vi "DBM inquiry.vi"(6 "컨트롤 참조":refnum<vi>[](array[refnum]), 7 "Query info":T2, 8 "에러 입력":errorcluster caption="에러 입력(에러 없음)", 11 "데이터":T1) -> (0 "에러 출력":errorcluster, 1 "None?":bool, 2 "Data":string[][](array[string]), 3 "테이블 참조 출력":refnum<vi>, 5 "데이터 out":T1)   [LabVIEW 2020]
uses:
  Controls/Clst_DBM data.ctl
  Controls/Clst_Query Info.ctl
  Controls/Cmd_Read Query.ctl
  <vilib>/addons/database/NI_Database_API.lvlib
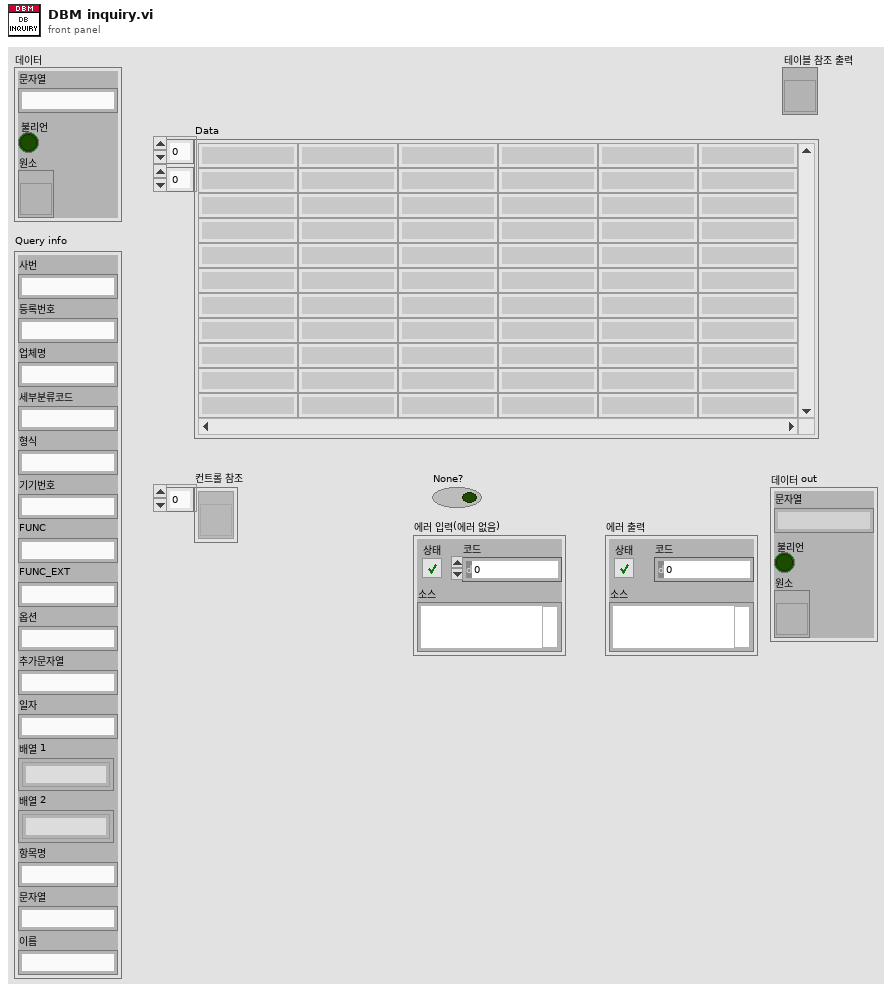
[diagram p1: front panel]
types:
  T1 = typedef "Clst_DBM data.ctl" = cluster{"문자열":string, "불리언":bool, "원소":refnum<vi>}
  T2 = typedef "Clst_Query Info.ctl" = cluster{"사번":string, "등록번호":string, "업체명":string, "세부분류코드":string, "형식":string, "기기번호":string, "FUNC":string, "FUNC_EXT":string, "옵션":string, "추가문자열":string, "일자":string, "배열 1":string[], "배열 2":string[], "항목명":string, "문자열":string, "이름":string}
  T3 = typedef "Cmd_Read Query.ctl" = enum16{"교정자 이름 얻기", "인증교정자 얻기", "기술책임자 얻기", "기책부책 얻기", "등록번호 얻기", "등록정보 얻기", "업체정보 얻기", "교정일자(CAMAS) 얻기", "교정일자(CALSTD) 얻기", "교정환경 얻기", "교정절차서 목록 얻기", "교정절차서명 얻기", "교정절차 목록얻기", "교정절차 얻기", "PROC 교정절차 얻기", "PROC SPEC 얻기", "교정절차(Func별) 얻기", "교정절차(Func_ext별) 얻기", "기관코드 얻기", "교정기능(세부분류) 얻기", "교정기능(모델) 얻기", "교정기능 목록 얻기", "교정기능 명칭 얻기", "교정기능 항목명칭 얻기", "DB (사용기준기) 얻기", "DB (기준기이름) 얻기", "DB (기준기이름목록) 얻기", "DB (기준기목록) 얻기", "DB (기준기값) 얻기", "DB (CMC) 얻기", "DB (FUNC) 얻기", "DB (CALNAME) 얻기", "DB (STDNAME) 얻기", "DB (SPEC) 얻기", "모델(항목전체) 얻기", "모델(최대범위) 얻기", "모델(최소범위) 얻기", "모델(최대최소) 얻기", "모델(범위조건) 얻기", "모델(등록요청) 얻기", "모델(형식별) 얻기", "모델(조건별) 얻기", "모델(모델검색) 얻기", "세부분류 목록 얻기", "기준기등록리스트 얻기", "STD Cal Date Check", "DB등록일자 얻기", "적용항목 얻기", "기타정보 얻기", "기준기요청 얻기", "서버버전 얻기"}
  T4 = typedef "NI_Database_API.lvlib/Conn ObjectReference.ctl" = refnum<k1>
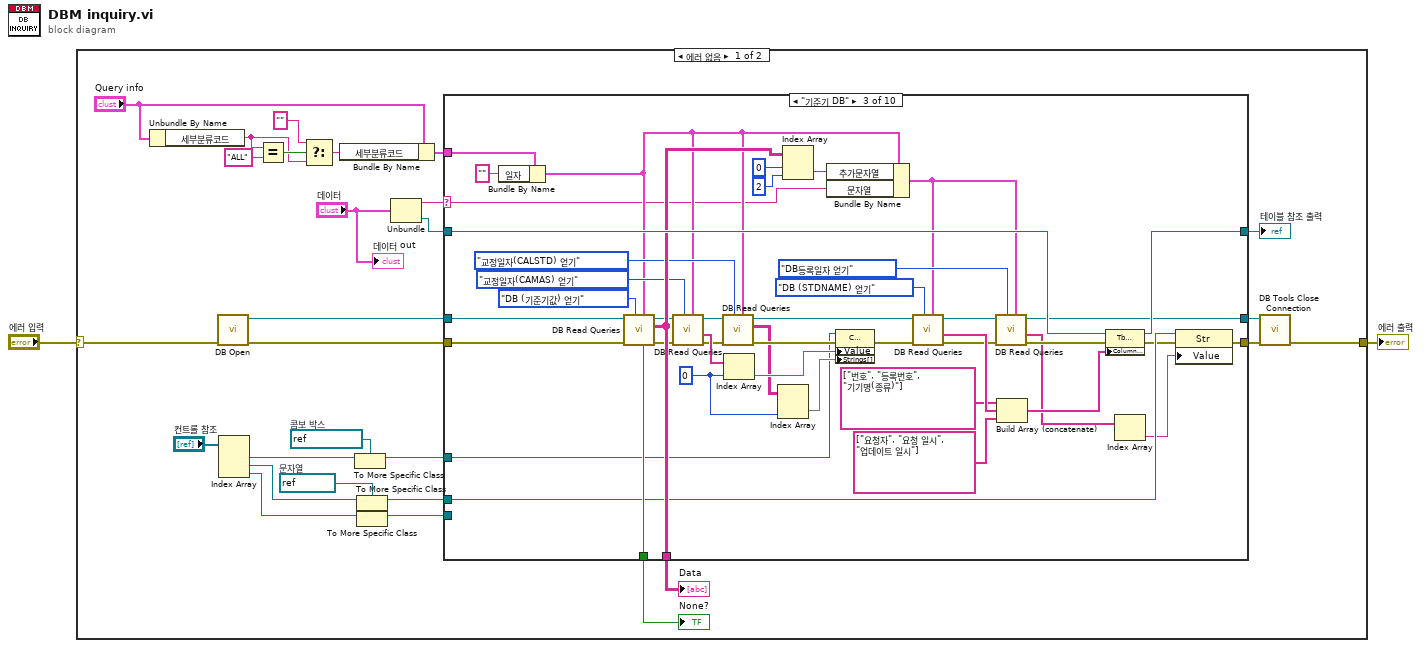
[diagram p0: block diagram]
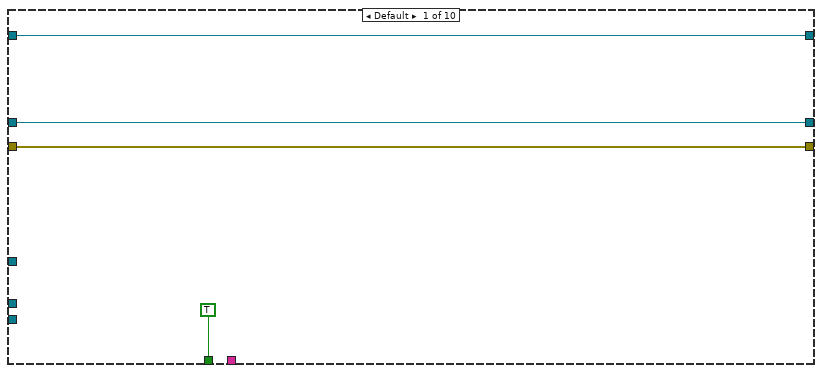
[diagram p2: hidden frame]
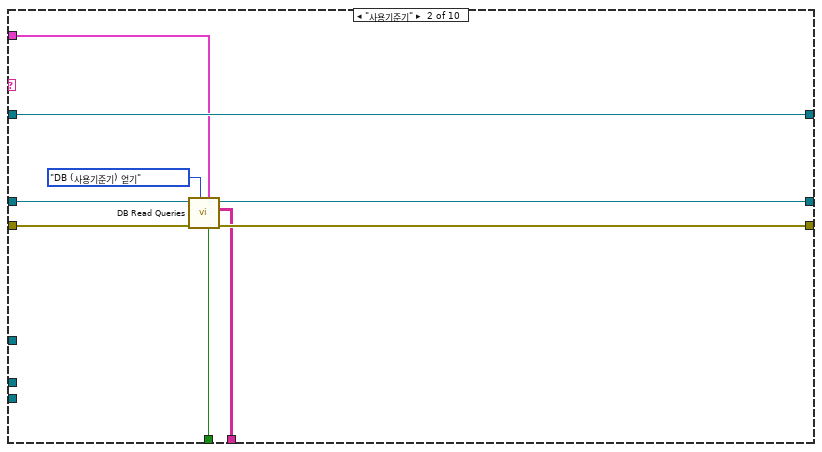
[diagram p3: hidden frame]
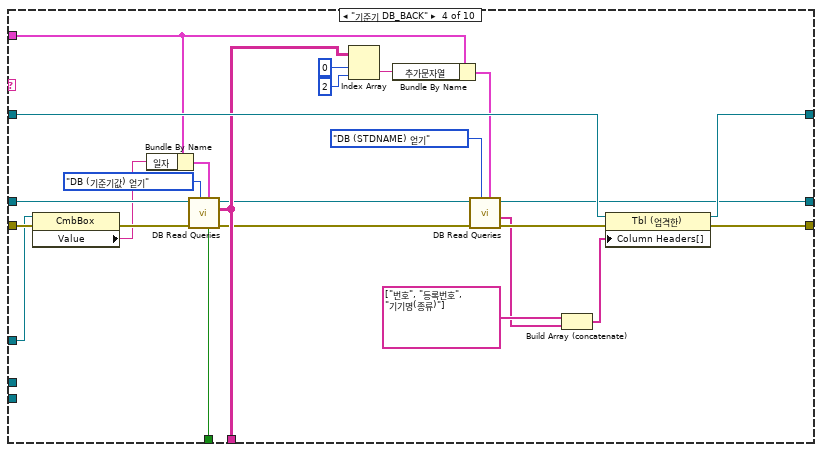
[diagram p4: hidden frame]
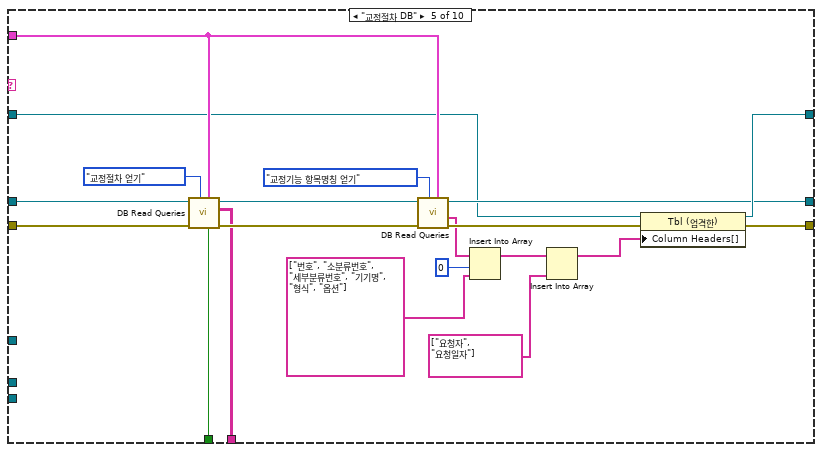
[diagram p5: hidden frame]
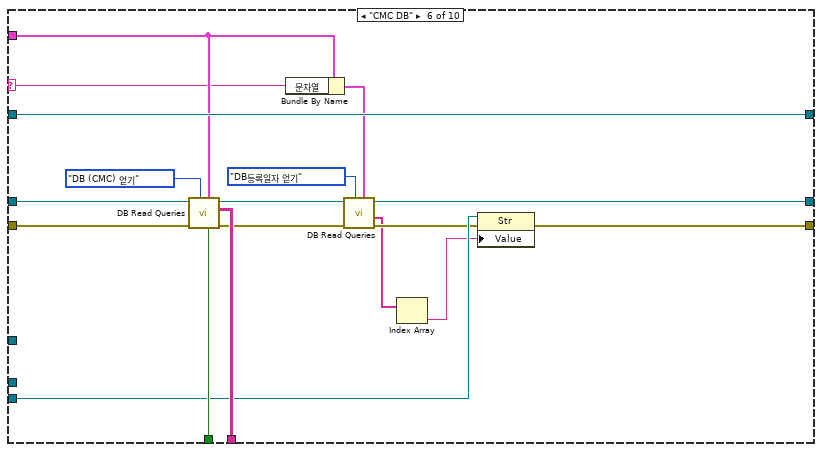
[diagram p6: hidden frame]
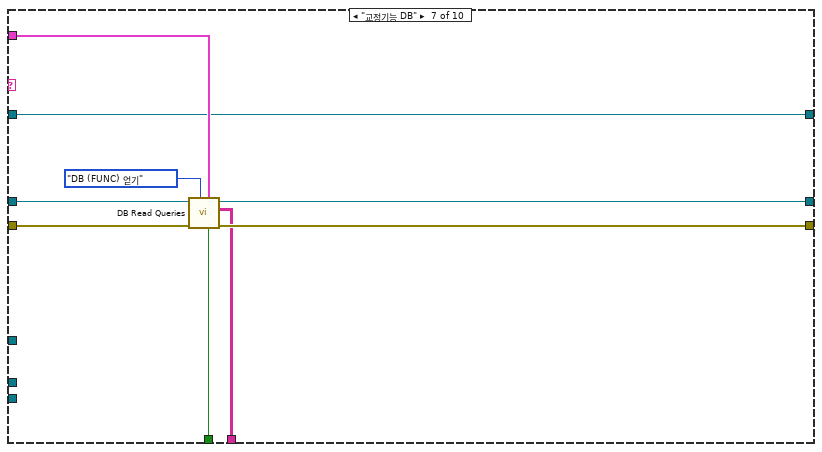
[diagram p7: hidden frame]
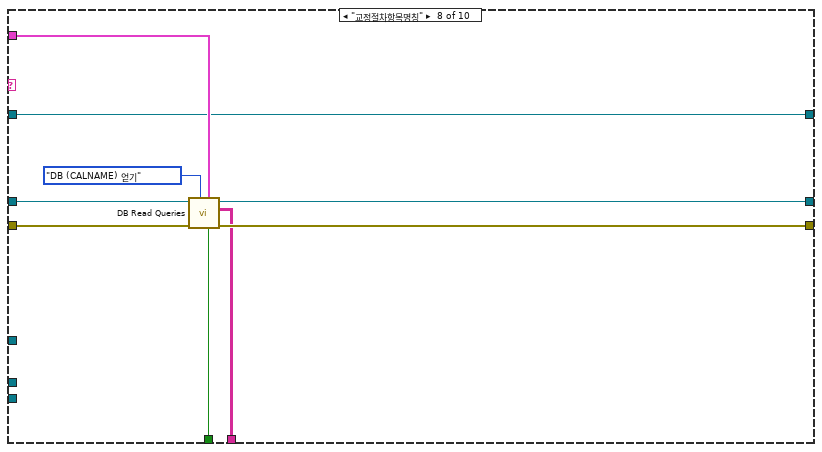
[diagram p8: hidden frame]
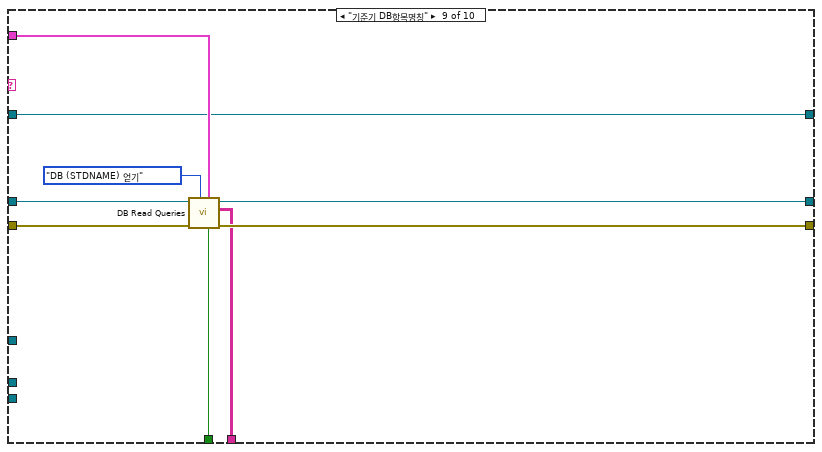
[diagram p9: hidden frame]
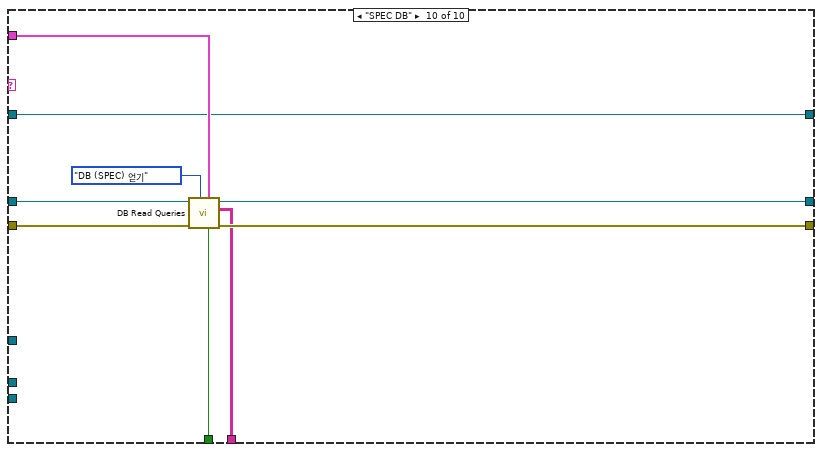
[diagram p10: hidden frame]
diagram:
  n1 = case shown="에러 없음" "에러 입력" {
    selector: "에러 입력" -> [w17 w187]
    tunnel: [w19 w187] -> w2
    frame No Error {
      w10 = refnum<vi> refnum  # 문자열
      w13 = refnum<vi> refnum  # 콤보 박스
      n2 = Unbundle By Name("Query info") -> ("세부분류코드"=w27:string)
      n3 = call "DB Open.vi"("에러 입력"=w17) -> ("에러 출력"=w22:errorcluster, "참조 번호 출력"=w21:T4)  [unwired: 9 in]
      n4 = Index Array(array="컨트롤 참조") -> (element #1=w15:refnum<vi>, element #2=w12:refnum<vi>, element #3=w9:refnum<vi>)  [unwired: 3 in]
      n5 = Equal?(x=w27, y="ALL") -> (x = y?=w28:bool)
      n6 = Select(t="", s=w28, f=w27) -> (s? t:f=w26:string)
      n7 = Bundle By Name(cluster="Query info", "세부분류코드"=w26) -> (w23:T2)
      n8 = To More Specific Class(target class=w13, reference=w15) -> (specific class reference=w14:refnum<vi>)  [unwired: 1 in, 1 out]
      n9 = To More Specific Class(target class=w10, reference=w12) -> (specific class reference=w11:refnum<vi>)  [unwired: 1 in, 1 out]
      n10 = To More Specific Class(target class=w10, reference=w9) -> (specific class reference=w8:refnum<vi>)  [unwired: 1 in, 1 out]
      n11 = Unbundle("데이터") -> ("문자열"=w5:string, "원소"=w3:refnum<vi>)  [unwired: 1 out]
      n12 = case shown="\"기준기 DB\"" w5 {
        selector: w5 -> [_ _ w46 _ _ w135 _ _ _ _]
        tunnel: [TRUE ("None?") w42 w87 w112 w131 w149 w158 w167 w176 w185] -> w30
        tunnel: w22 -> [w34 w41 w86 w92 w130 w148 w157 w166 w175 w184]
        tunnel: [w34 w40 w47 w111 w128 w143 w156 w165 w174 w183] -> w20
        tunnel: [_ w39 w81 w103 w127 w147 w155 w164 w173 w182] -> w24
        tunnel: [w32 w37 w85 w110 w126 w146 w152 w161 w170 w179] -> w7
        tunnel: w23 -> [_ w35 w60 w94 w124 w137 w154 w163 w172 w181]
        tunnel: [w33 w38 w54 w107 w123 w139 w153 w162 w171 w180] -> w18
        tunnel: w3 -> [w32 w37 w84 w109 w122 w146 w152 w161 w170 w179]
        tunnel: w21 -> [w33 w36 w83 w108 w121 w145 w151 w160 w169 w178]
        tunnel: w14 -> [_ _ w50 w90 _ _ _ _ _ _]
        tunnel: w11 -> [_ _ w49 _ _ _ _ _ _ _]
        tunnel: w8 -> [_ _ _ _ _ w144 _ _ _ _]
        frame Default {
        }
        frame "사용기준기" {
          n13 = call "DB Read Queries.vi"("Query info"=w35, "Query Command"=Cmd_Read_Query."DB (사용기준기) 얻기", "에러 입력(에러 없음)"=w41, "참조 번호 입력"=w36) -> ("에러 출력"=w40:errorcluster, "Data"=w39:string[][], "참조 번호 출력"=w38:T4, "None?"=w42:bool)  [unwired: 3 in, 1 out]
        }
        frame "기준기 DB" {
          w62 = 0 ("인덱스 (행)")
          n14 = Bundle By Name(cluster=w60, "일자"="") -> (w58:T2)
          n15 = call "DB Read Queries.vi"("Query info"=w58, "Query Command"=Cmd_Read_Query."DB (기준기값) 얻기", "에러 입력(에러 없음)"=w86, "참조 번호 입력"=w83) -> ("에러 출력"=w75:errorcluster, "Data"=w81:string[][], "참조 번호 출력"=w76:T4, "None?"=w87:bool)  [unwired: 3 in, 1 out]
          n16 = call "DB Read Queries.vi"("Query info"=w58, "Query Command"=Cmd_Read_Query."교정일자(CAMAS) 얻기", "에러 입력(에러 없음)"=w75, "참조 번호 입력"=w76) -> ("에러 출력"=w68:errorcluster, "Data (0번행)"=w74:string[], "참조 번호 출력"=w66:T4)  [unwired: 3 in, 2 out]
          n17 = call "DB Read Queries.vi"("Query info"=w58, "Query Command"=Cmd_Read_Query."교정일자(CALSTD) 얻기", "에러 입력(에러 없음)"=w68, "참조 번호 입력"=w66) -> ("에러 출력"=w67:errorcluster, "Data"=w63:string[][], "참조 번호 출력"=w65:T4)  [unwired: 3 in, 2 out]
          n18 = Index Array(array=w74, index=w62) -> (element=w71:string)
          n19 = Index Array(array=w63, index (col)=w62) -> (element=w61:string[])  [unwired: 1 in]
          n20 = Index Array(array=w81, index (row)=0 ("인덱스 (행)"), index (col)=2 ("비활성화된 인덱스 (열)")) -> (element=w78:string)
          n21 = Bundle By Name(cluster=w58, "추가문자열"=w78, "문자열"=w46) -> (w52:T2)
          n22 = property class="CmbBox"(reference=w50, error in=w67, "Value"=w71, "Strings[]"=w61) -> (error out=w72:errorcluster)  [unwired: 1 out]
          n23 = call "DB Read Queries.vi"("Query info"=w52, "Query Command"=Cmd_Read_Query."DB (STDNAME) 얻기", "에러 입력(에러 없음)"=w72, "참조 번호 입력"=w65) -> ("에러 출력"=w56:errorcluster, "Data (0번행)"=w77:string[], "참조 번호 출력"=w57:T4)  [unwired: 3 in, 2 out]
          n24 = call "DB Read Queries.vi"("Query info"=w52, "Query Command"=Cmd_Read_Query."DB등록일자 얻기", "에러 입력(에러 없음)"=w56, "참조 번호 입력"=w57) -> ("에러 출력"=w55:errorcluster, "Data (0번행)"=w51:string[], "참조 번호 출력"=w54:T4)  [unwired: 3 in, 2 out]
          n25 = Build Array (concatenate)(string[] ["번호", "등록번호", "기기명(종류)"], w77, string[] ["요청자", "요청 일시", "업데이트 일시"]) -> (w70:string[])
          n26 = property class="Tbl (엄격한)"(reference=w84, error in=w55, "Column Headers[]"=w70) -> (reference out=w85:refnum<vi>, error out=w48:errorcluster)
          n27 = Index Array(array=w51) -> (element=w45:string)  [unwired: 1 in]
          n28 = property class="Str"(reference=w49, error in=w48, "Value"=w45) -> (error out=w47:errorcluster)  [unwired: 1 out]
        }
        frame "기준기 DB_BACK" {
          n29 = property class="CmbBox"(reference=w90, error in=w92) -> (error out=w91:errorcluster, "Value"=w89:string)  [unwired: 1 out]
          n30 = Bundle By Name(cluster=w94, "일자"=w89) -> (w93:T2)
          n31 = call "DB Read Queries.vi"("Query info"=w93, "Query Command"=Cmd_Read_Query."DB (기준기값) 얻기", "에러 입력(에러 없음)"=w91, "참조 번호 입력"=w108) -> ("에러 출력"=w97:errorcluster, "Data"=w103:string[][], "참조 번호 출력"=w96:T4, "None?"=w112:bool)  [unwired: 3 in, 1 out]
          n32 = Index Array(array=w103, index (row)=0 ("인덱스 (행)"), index (col)=2 ("비활성화된 인덱스 (열)")) -> (element=w100:string)
          n33 = Bundle By Name(cluster=w94, "추가문자열"=w100) -> (w104:T2)
          n34 = call "DB Read Queries.vi"("Query info"=w104, "Query Command"=Cmd_Read_Query."DB (STDNAME) 얻기", "에러 입력(에러 없음)"=w97, "참조 번호 입력"=w96) -> ("에러 출력"=w106:errorcluster, "Data (0번행)"=w95:string[], "참조 번호 출력"=w107:T4)  [unwired: 3 in, 2 out]
          n35 = Build Array (concatenate)(string[] ["번호", "등록번호", "기기명(종류)"], w95) -> (w99:string[])
          n36 = property class="Tbl (엄격한)"(reference=w109, error in=w106, "Column Headers[]"=w99) -> (reference out=w110:refnum<vi>, error out=w111:errorcluster)
        }
        frame "교정절차 DB" {
          n37 = call "DB Read Queries.vi"("Query info"=w124, "Query Command"=Cmd_Read_Query."교정절차 얻기", "에러 입력(에러 없음)"=w130, "참조 번호 입력"=w121) -> ("에러 출력"=w129:errorcluster, "Data"=w127:string[][], "참조 번호 출력"=w125:T4, "None?"=w131:bool)  [unwired: 3 in, 1 out]
          n38 = call "DB Read Queries.vi"("Query info"=w124, "Query Command"=Cmd_Read_Query."교정기능 항목명칭 얻기", "에러 입력(에러 없음)"=w129, "참조 번호 입력"=w125) -> ("Data (0번행)"=w119:string[], "참조 번호 출력"=w123:T4)  [unwired: 3 in, 3 out]
          n39 = Insert Into Array(array=w119, index=0 ("인덱스"), new element=string[] ["번호", "소분류번호", "세부분류번호", "기기명", "형식", "옵션"]) -> (w116:string[])
          n40 = Insert Into Array(array=w116, new element=string[] ["요청자", "요청일자"]) -> (w115:string[])  [unwired: 1 in]
          n41 = property class="Tbl (엄격한)"(reference=w122, error in=w129, "Column Headers[]"=w115) -> (reference out=w126:refnum<vi>, error out=w128:errorcluster)
        }
        frame "CMC DB" {
          n42 = call "DB Read Queries.vi"("Query info"=w137, "Query Command"=Cmd_Read_Query."DB (CMC) 얻기", "에러 입력(에러 없음)"=w148, "참조 번호 입력"=w145) -> ("에러 출력"=w142:errorcluster, "Data"=w147:string[][], "참조 번호 출력"=w140:T4, "None?"=w149:bool)  [unwired: 3 in, 1 out]
          n43 = Bundle By Name(cluster=w137, "문자열"=w135) -> (w136:T2)
          n44 = call "DB Read Queries.vi"("Query info"=w136, "Query Command"=Cmd_Read_Query."DB등록일자 얻기", "에러 입력(에러 없음)"=w142, "참조 번호 입력"=w140) -> ("에러 출력"=w141:errorcluster, "Data (0번행)"=w134:string[], "참조 번호 출력"=w139:T4)  [unwired: 3 in, 2 out]
          n45 = Index Array(array=w134) -> (element=w133:string)  [unwired: 1 in]
          n46 = property class="Str"(reference=w144, error in=w141, "Value"=w133) -> (error out=w143:errorcluster)  [unwired: 1 out]
        }
        frame "교정기능 DB" {
          n47 = call "DB Read Queries.vi"("Query info"=w154, "Query Command"=Cmd_Read_Query."DB (FUNC) 얻기", "에러 입력(에러 없음)"=w157, "참조 번호 입력"=w151) -> ("에러 출력"=w156:errorcluster, "Data"=w155:string[][], "참조 번호 출력"=w153:T4, "None?"=w158:bool)  [unwired: 3 in, 1 out]
        }
        frame "교정절차항목명칭" {
          n48 = call "DB Read Queries.vi"("Query info"=w163, "Query Command"=Cmd_Read_Query."DB (CALNAME) 얻기", "에러 입력(에러 없음)"=w166, "참조 번호 입력"=w160) -> ("에러 출력"=w165:errorcluster, "Data"=w164:string[][], "참조 번호 출력"=w162:T4, "None?"=w167:bool)  [unwired: 3 in, 1 out]
        }
        frame "기준기 DB항목명칭" {
          n49 = call "DB Read Queries.vi"("Query info"=w172, "Query Command"=Cmd_Read_Query."DB (STDNAME) 얻기", "에러 입력(에러 없음)"=w175, "참조 번호 입력"=w169) -> ("에러 출력"=w174:errorcluster, "Data"=w173:string[][], "참조 번호 출력"=w171:T4, "None?"=w176:bool)  [unwired: 3 in, 1 out]
        }
        frame "SPEC DB" {
          n50 = call "DB Read Queries.vi"("Query info"=w181, "Query Command"=Cmd_Read_Query."DB (SPEC) 얻기", "에러 입력(에러 없음)"=w184, "참조 번호 입력"=w178) -> ("에러 출력"=w183:errorcluster, "Data"=w182:string[][], "참조 번호 출력"=w180:T4, "None?"=w185:bool)  [unwired: 3 in, 1 out]
        }
      }
      "Data" <- w24
      "None?" <- w30
      "테이블 참조 출력" <- w7
      n51 = call <vilib>:"DB Tools Close Connection.vi"("error in (no error)"=w20, "connection reference"=w18) -> ("error out"=w19:errorcluster)  [unwired: 5 in]
      "데이터 out" <- "데이터"
    }
    frame Error {
    }
  }
  "에러 출력" <- w2
